vi "Create Sysdef Tree from Parameters Clusters.vi"(8 "error in":errorcluster, 10 "Channels":T1[](array[typedef]), 11 "Device Ptr":u64) -> (0 "error out":errorcluster, 3 "Device Ptr dup":u64)   [LabVIEW 2019, in "Ballard Arinc-429 System Explorer.lvlib"]
uses:
  Ballard Arinc-429 System Explorer.lvlib
  Parse Parameters File/XML_Channel.ctl
  Parse Parameters File/XML_Label.ctl
  Parse Parameters File/XML_Parameter.ctl
  Shared/Controls and Global/Global.vi
  <vilib>/NI VeriStand/Custom Device Tools/Custom Device Utility Library/NI VeriStand - Search for Item by GUID.vi
  <vilib>/NI VeriStand/Custom Device Tools/Custom Device Utility Library/NI VeriStand - Search for All Items by GUID.vi
  <vilib>/NI VeriStand/Custom Device API/NI VeriStand - Get Item Property.vi
  <vilib>/NI VeriStand/Custom Device API/Get Item Property (U16).vi
  <vilib>/NI VeriStand/Custom Device API/NI VeriStand - Get Item Children.vi
  <vilib>/NI VeriStand/Custom Device API/Get Item Property (U32).vi
  <vilib>/NI VeriStand/Custom Device API/Get Item Property (Boolean).vi
  Shared/Ballard Arinc-429 Shared.lvlib
  <vilib>/NI VeriStand/Custom Device Tools/Custom Device Utility Library/Custom Device Utility Library.lvlib
  <vilib>/NI VeriStand/Custom Device API/Custom Device API.lvlib
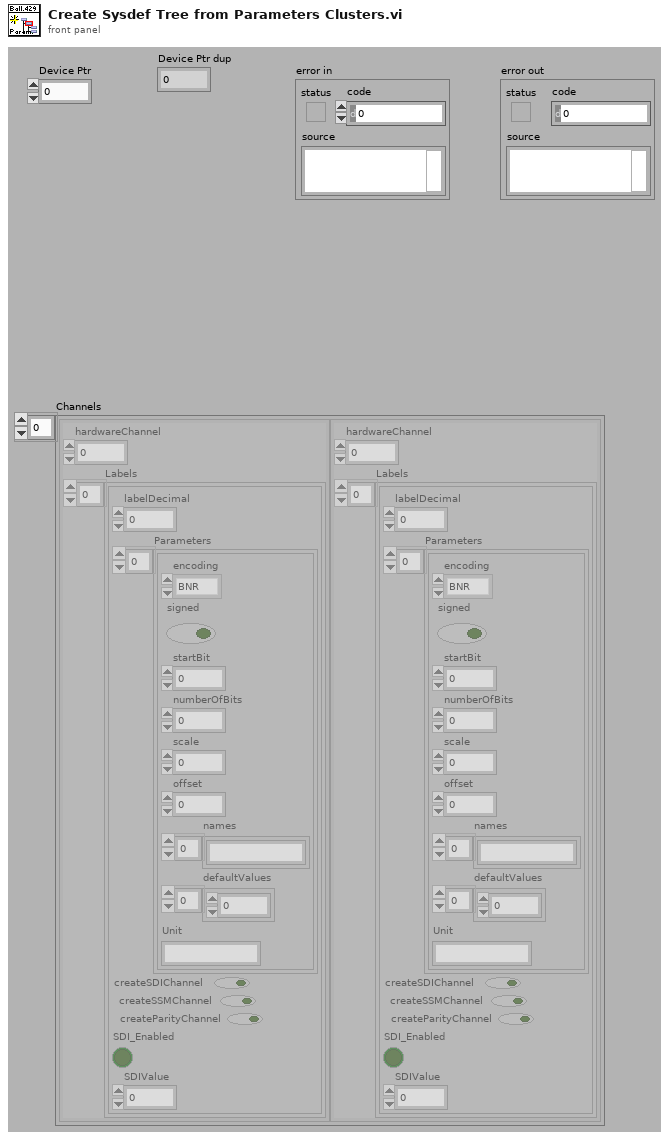
[diagram p1: front panel]
types:
  T1 = typedef "XML_Channel.ctl" = cluster{"hardwareChannel":i32, "Labels":T2[]}
  T2 = typedef "XML_Label.ctl" = cluster{"labelDecimal":i32, "Parameters":T3[], "createSDIChannel":bool, "createSSMChannel":bool, "createParityChannel":bool, "SDI_Enabled":bool, "SDIValue":u8}
  T3 = typedef "XML_Parameter.ctl" = cluster{"encoding":enum16{"BNR", "BCD", "Discrete"}, "signed":bool, "startBit":i32, "numberOfBits":i32, "scale":dbl, "offset":dbl, "names":string[], "defaultValues":dbl[], "Unit":string}
  T4 = typedef "Custom Device API.lvlib/Custom Device Item Ref.ctl" = u64
  T5 = typedef "Custom Device API.lvlib/Custom Device Item Info.ctl" = cluster{"Name":string, "Is Channel":bool, "GUID":string, "Is Waveform":bool}
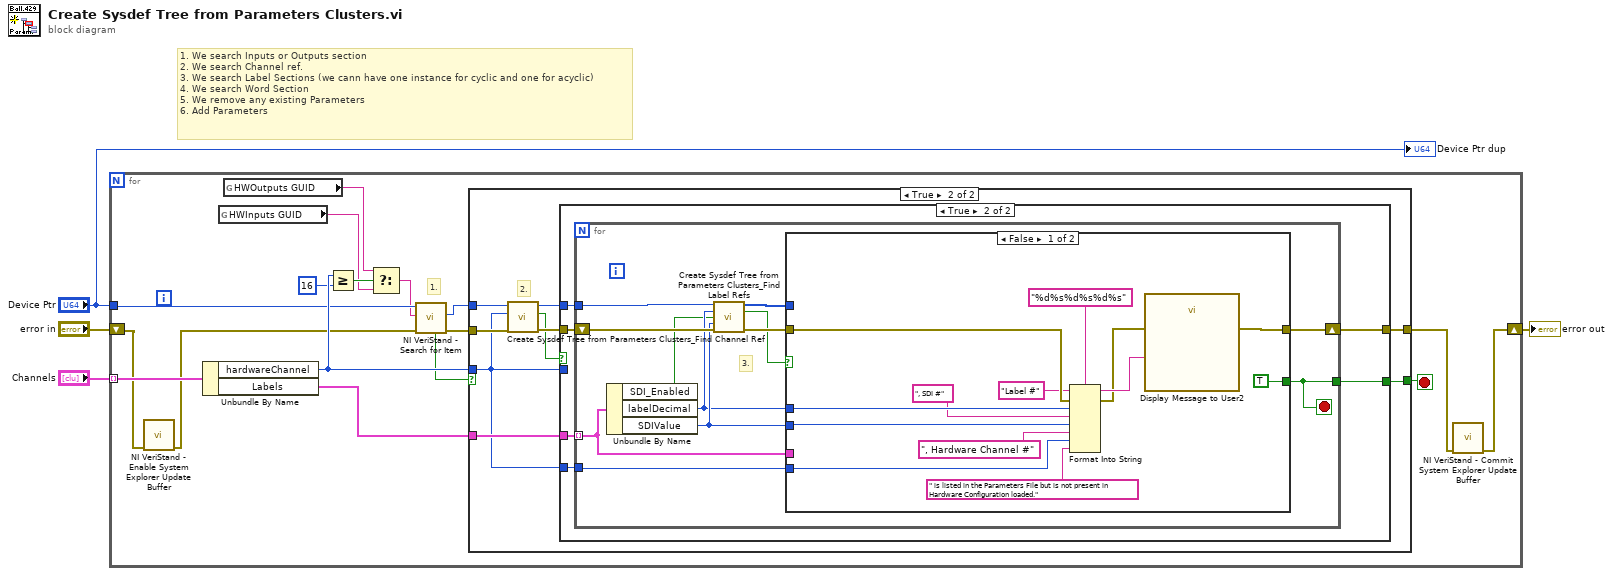
[diagram p0: block diagram]
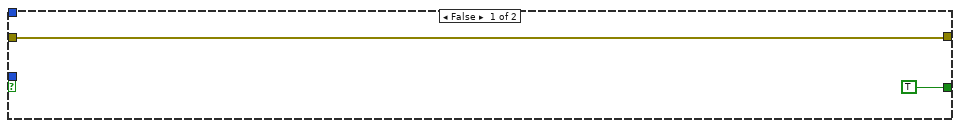
[diagram p2: hidden frame]
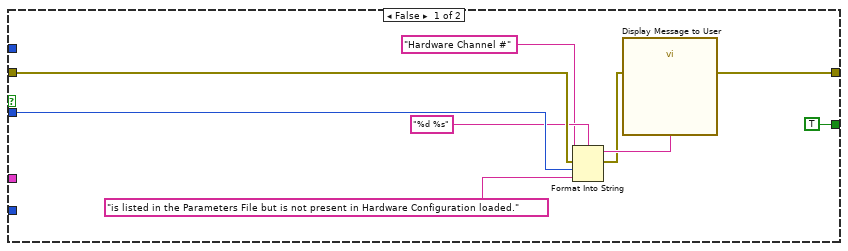
[diagram p3: hidden frame]
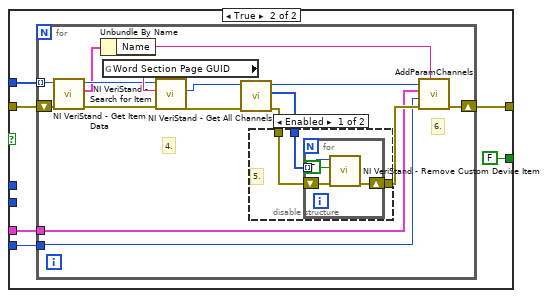
[diagram p4: hidden frame]
diagram:
  # "1. We search Inputs or Outputs section\n2. We search Channel ref.\n3. We search Label Sections (we cann have one instance for cyclic and one for acyclic)\n4. We search Word Section\n5. We remove any existing Parameters\n6. Add Parameters"
  n1 = for {
    tunnel: "Device Ptr" -> [w16]
    shift-right: [w5] -> w2
    shift-left: "error in" -> [w8]
    tunnel: "Channels" -> [w21] mode=indexing
    stop <- w9 stop-if-true
    # "1."
    n2 = call <vilib>:"NI VeriStand - Enable System Explorer Update Buffer.vi"("error in (no error)"=w8) -> ("error out"=w7:errorcluster)  [unwired: 10 in]
    n3 = Unbundle By Name(w21) -> ("hardwareChannel"=w19:i32, "Labels"=w20:T2[])
    n4 = global read "Global.vi" "HWInputs GUID"() -> (w11:string)
    n5 = global read "Global.vi" "HWOutputs GUID"() -> (w12:string)
    n6 = Greater Or Equal?(x=w19, y=16) -> (x >= y?=w17:bool)
    n7 = Select(t=w12, s=w17, f=w11) -> (s? t:f=w10:string)
    n8 = call-poly <vilib>:"NI VeriStand - Search for Item.vi"("error in"=w7, "Item GUID"=w10, "Section Ref in"=w16) -> ("error out"=w13:errorcluster, "Item Ref"=w15:T4, "Found"=w14:bool)  [unwired: 5 in, 1 out]
    n9 = case shown="True" w14 {
      tunnel: [w23 w32] -> w6
      tunnel: w20 -> [_ w29]
      tunnel: w19 -> [_ w25]
      tunnel: w15 -> [_ w24]
      tunnel: w13 -> [w23 w27]
      tunnel: [TRUE w26] -> w9
      frame False {
      }
      frame True {
        # "2."
        n10 = call "Create Sysdef Tree from Parameters Clusters_Find Channel Ref.vi"("error in (no error)"=w27, "hardwareChannel"=w25, "Item Ref in"=w24) -> ("error out"=w31:errorcluster, "Found"=w30:bool, "Item Ref out"=w28:T4)  [unwired: 6 in]
        n11 = case shown="True" w30 {
          tunnel: [w41 w45] -> w32
          tunnel: w31 -> [w40 w47]
          tunnel: w28 -> [_ w42]
          tunnel: w25 -> [w37 _]
          tunnel: w29 -> [_ w46]
          tunnel: w25 -> [_ w44]
          tunnel: [TRUE w43] -> w26
          frame False {
            n12 = Format Into String(format string="%d %s", initial string="Hardware Channel #", error in=w40, w37, "is listed in the Parameters File but is not present in Hardware Configuration loaded." ("initial string")) -> (resulting string=w39:string, error out=w38:errorcluster)
            n13 = call "Display Message to User"("error in (no error)"=w38, "Message"=w39) -> ("error out"=w41:errorcluster)  [unwired: 8 in, 1 out]
          }
          frame True {
            n14 = for {
              tunnel: w42 -> [w56]
              tunnel: w46 -> [w58] mode=indexing
              shift-right: [w59] -> w45
              shift-left: w47 -> [w55]
              tunnel: w44 -> [w51]
              tunnel: [w57] -> w43
              stop <- w57 stop-if-true
              # "3."
              n15 = Unbundle By Name(w58) -> ("SDI_Enabled"=w48:bool, "labelDecimal"=w49:i32, "SDIValue"=w50:u8)
              n16 = call "Create Sysdef Tree from Parameters Clusters_Find Label Refs.vi"("Item Ref in"=w56, "decimalLabel"=w49, "SDI_Enabled"=w48, "SDIValue"=w50, "error in (no error)"=w55) -> ("Array of Refs"=w53:T4[], "Found"=w52:bool, "error out"=w54:errorcluster)  [unwired: 8 in]
              n17 = case shown="False" w52 {
                tunnel: w54 -> [w70 w76]
                tunnel: w53 -> [_ w74]
                tunnel: [w71 w78] -> w59
                tunnel: w58 -> [_ w77]
                tunnel: w49 -> [w72 _]
                tunnel: [TRUE FALSE] -> w57
                tunnel: w51 -> [w63 w73]
                tunnel: w50 -> [w61 _]
                frame False {
                  n18 = Format Into String(format string="%d%s%d%s%d%s", initial string="Label #", error in=w70, w72, ", SDI #" ("initial string"), w61, ", Hardware Channel #" ("initial string"), w63, " is listed in the Parameters File but is not present in Hardware Configuration loaded." ("initial string")) -> (resulting string=w66:string, error out=w65:errorcluster)
                  n19 = call "Display Message to User2"("error in (no error)"=w65, "Message"=w66) -> ("error out"=w71:errorcluster)  [unwired: 8 in, 1 out]
                }
                frame True {
                  n20 = for {
                    tunnel: w77 -> [w86]
                    tunnel: w74 -> [w80] mode=indexing
                    shift-right: [w87] -> w78
                    shift-left: w76 -> [w85]
                    tunnel: w73 -> [w79]
                    # "6."
                    # "4."
                    n21 = call <vilib>:"NI VeriStand - Get Item Data.vi"("error in (no error)"=w85, "Item Ref in"=w80) -> ("error out"=w83:errorcluster, "Item Info"=w82:T5, "Item Ref out"=w84:T4)  [unwired: 6 in, 1 out]
                    n22 = Unbundle By Name(w82) -> ("Name"=w81:string)
                    n23 = global read "Global.vi" "Word Section Page GUID"() -> (w94:string)
                    n24 = call-poly <vilib>:"NI VeriStand - Search for Item.vi"("error in"=w83, "Item GUID"=w94, "Section Ref in"=w84) -> ("error out"=w92:errorcluster, "Item Ref"=w93:T4)  [unwired: 5 in, 2 out]
                    n25 = call <vilib>:"NI VeriStand - Get All Channels.vi"("error in"=w92, "Section Ref in"=w93) -> ("error out"=w90:errorcluster, "Channel Refs"=w91:T4[], "Section Ref out"=w89:T4)  [unwired: 6 in, 1 out]
                    n26 = disable-structure shown="Enabled" {
                      disable-tunnel: w91 -> [w97 _]
                      disable-tunnel: w90 -> [w96 w102]
                      disable-tunnel: [w95 w102] -> w88
                      frame Enabled {
                        # "5."
                        n27 = for {
                          tunnel: w97 -> [w101] mode=indexing
                          shift-right: [w99] -> w95
                          shift-left: w96 -> [w100]
                          n28 = call <vilib>:"NI VeriStand - Remove Custom Device Item.vi"("error in (no error)"=w100, "Force Delete (F)"=TRUE, "Item Ref in"=w101) -> ("error out"=w99:errorcluster)  [unwired: 7 in, 1 out]
                        }
                      }
                      frame Disabled {
                      }
                    }
                    n29 = call "AddParamChannels.vi"("Label Name"=w81, "error in"=w88, "HardwareChannel"=w79, "Label Parameters"=w86, "Node Ref In"=w89) -> ("error out"=w87:errorcluster)  [unwired: 5 in, 1 out]
                  }
                }
              }
            }
          }
        }
      }
    }
    n30 = call <vilib>:"NI VeriStand - Commit System Explorer Update Buffer.vi"("error in (no error)"=w6) -> ("error out"=w5:errorcluster)  [unwired: 10 in]
  }
  "error out" <- w2
  "Device Ptr dup" <- "Device Ptr"
